vi "AdvancedComparisonFunctions1.vi"() -> ()   [LabVIEW 2020]
panel:
  out "x = y?":bool[](array[boolean])
  in  "element 8":dbl
  in  "element 7":dbl
  in  "element 6":dbl
  in  "element 5":dbl
  in  "element 4":dbl
  in  "element 3":dbl
  in  "element 2":dbl
  in  "element":dbl
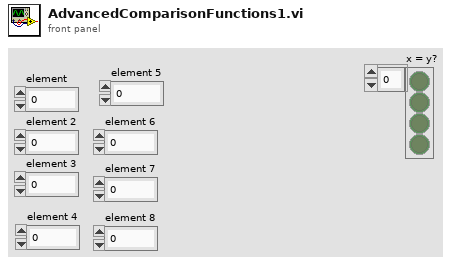
[diagram p1: front panel]
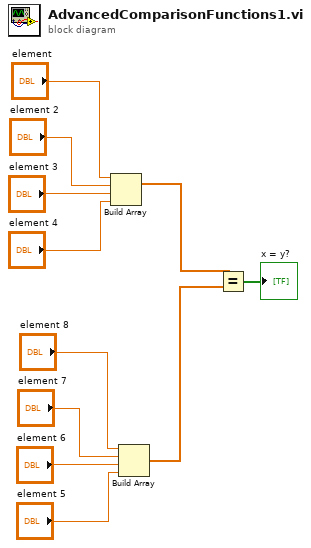
[diagram p0: block diagram]
diagram:
  n1 = Build Array("element", "element 2", "element 3", "element 4") -> (w3:dbl[])
  n2 = Build Array("element 8", "element 7", "element 6", "element 5") -> (w2:dbl[])
  n3 = Equal?(x=w3, y=w2) -> (x = y?=→"x = y?":bool[])
